vi "FisherPaykel Send Command.vi"(7 "Debug":bool, 8 "error in (no error)":errorcluster, 10 "Send Command":string, 11 "VISA Refnum in":refnum<visa-resource-name>) -> (0 "error out":errorcluster, 2 "Command (Debug)":string, 3 "VISA Refnum out":refnum<visa-resource-name>)   [LabVIEW 2016]
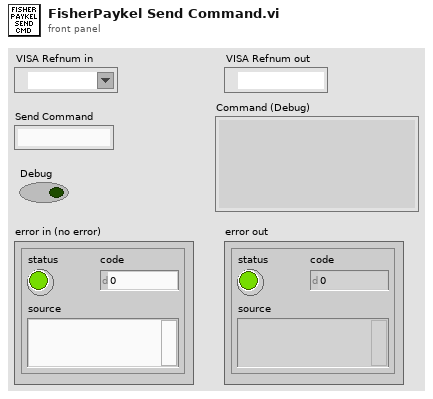
[diagram p1: front panel]
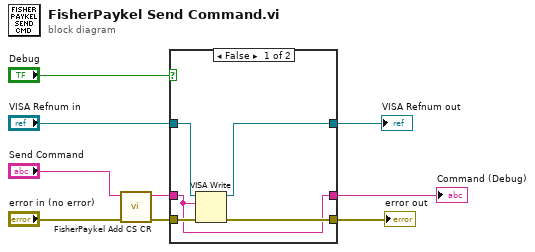
[diagram p0: block diagram]
diagram:
  n1 = call "FisherPaykel Add CS CR.vi"("Error In"="error in (no error)", "Command Input"="Send Command") -> ("Error Out"=w9:errorcluster, "Command w/ [CS] [CR]"=w2:string)  [unwired: 8 in]
  n2 = case shown="False" "Debug" {
    tunnel: w2 -> [w10 w15]
    tunnel: "VISA Refnum in" -> [w14 w16]
    tunnel: w9 -> [w13 w17]
    tunnel: [w12 w17] -> w5
    tunnel: [w11 w16] -> w6
    tunnel: [w10 w15] -> w1
    frame False {
      n3 = VISA Write(VISA resource name=w14, write buffer=w10, error in (no error)=w13) -> (VISA resource name out=w11:refnum<visa-resource-name>, error out=w12:errorcluster)  [unwired: 1 out]
    }
    frame True {
    }
  }
  "error out" <- w5
  "VISA Refnum out" <- w6
  "Command (Debug)" <- w1
